vi "invert.vi"(8 "error in (no error)":errorcluster, 10 "Invert":bool, 11 "Refnum in":T1) -> (0 "error out":errorcluster, 2 "Array_out":u8[][](array[numeric]))   [LabVIEW 2019, in "Lib_Simx.lvlib"]
doc: "Inverts the mask and create pixels array"
uses:
  <vilib>/vision/Image Controls.llb/IMAQ Image.ctl
  Lib_Simx.lvlib
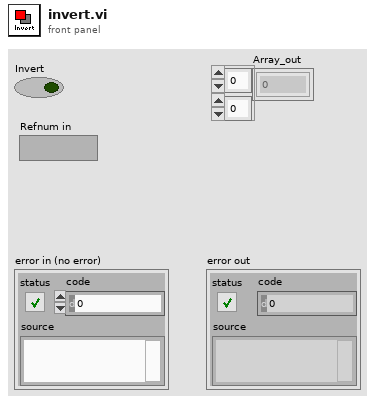
[diagram p1: front panel]
types:
  T1 = typedef "IMAQ Image.ctl" = refnum<image>
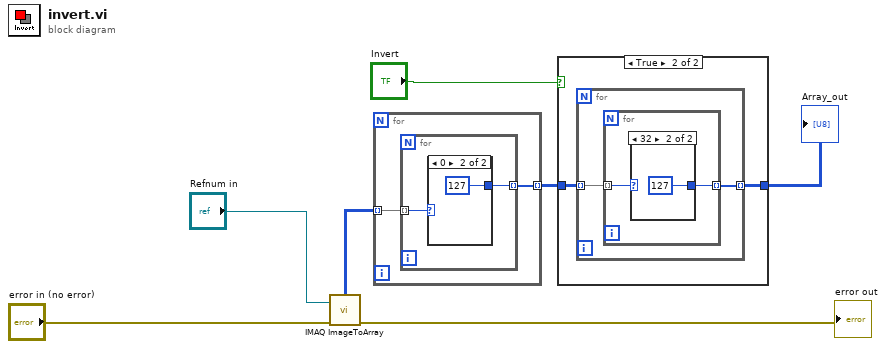
[diagram p0: block diagram]
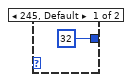
[diagram p2: hidden frame]
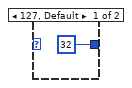
[diagram p4: hidden frame]
diagram:
  n1 = call "IMAQ ImageToArray"("error in (no error)"="error in (no error)", "Image"="Refnum in") -> ("error out"=→"error out":errorcluster, "Image Pixels (U8)"=w6:u8[][])  [unwired: 2 in, 3 out]
  n2 = for {
    tunnel: w6 -> [w9] mode=indexing
    tunnel: [w8] -> w5 mode=indexing
    n3 = for {
      tunnel: w9 -> [w11] mode=indexing
      tunnel: [w10] -> w8 mode=indexing
      n4 = case shown="0" w11 {
        tunnel: [u8 32 u8 127] -> w10
        frame 245, Default {
        }
        frame 0 {
        }
      }
    }
  }
  n5 = case shown="True" "Invert" {
    tunnel: w5 -> [w14 w16]
    tunnel: [w14 w15] -> w3
    frame False {
    }
    frame True {
      n6 = for {
        tunnel: [w18] -> w15 mode=indexing
        tunnel: w16 -> [w17] mode=indexing
        n7 = for {
          tunnel: [w20] -> w18 mode=indexing
          tunnel: w17 -> [w19] mode=indexing
          n8 = case shown="32" w19 {
            tunnel: [u8 32 u8 127] -> w20
            frame 127, Default {
            }
            frame 32 {
            }
          }
        }
      }
    }
  }
  "Array_out" <- w3
